vi "Blank Module Data (Constant).vi"() -> (0 "Blank Module Data":T1)   [LabVIEW 2023, in "Error Manager.lvlib" / "New Error Dialogue GUI.lvlib"]
doc: "Outputs a \"blank\" Module Data cluster. Use this to initialise the Module Data, or to reset or clear it.\n\n\"blank\" is used to mean default, empty or initial values."
uses:
  New Error Dialogue GUI.lvlib
  Module Data (cluster).ctl
  Module Data - Inputs (cluster).ctl
  Module Data - Work (cluster).ctl
  Module Data - Outputs (cluster).ctl
panel:
  # "Development\ncontrols/indicators useful for development and testing, but which are not outputs of the VI"
  # "Input\nInputs to the VI"
  # "Output\nOutputs of the VI"
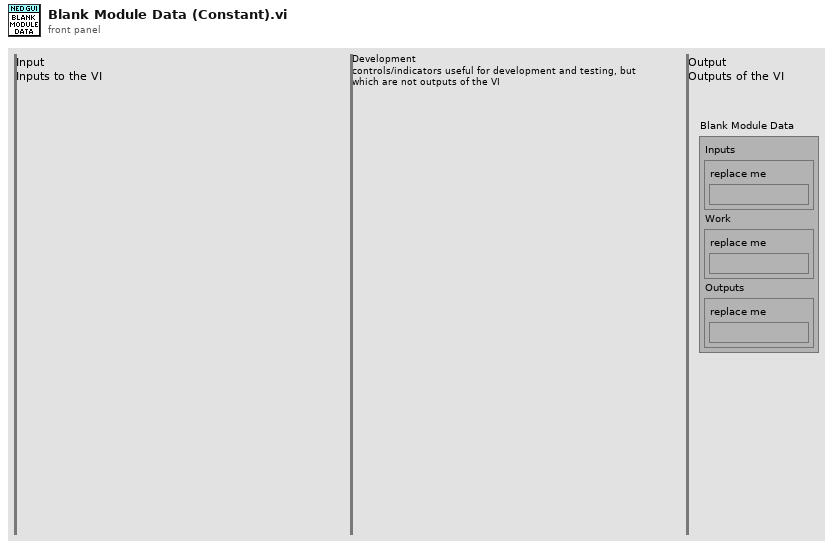
[diagram p1: front panel]
types:
  T1 = typedef "Error Manager.lvlib/New Error Dialogue GUI.lvlib/Module Data (cluster).ctl" = cluster{"Inputs":T2, "Work":T3, "Outputs":T4}
  T2 = typedef "Error Manager.lvlib/New Error Dialogue GUI.lvlib/Module Data - Inputs (cluster).ctl" = cluster{"replace me":string}
  T3 = typedef "Error Manager.lvlib/New Error Dialogue GUI.lvlib/Module Data - Work (cluster).ctl" = cluster{"replace me":string}
  T4 = typedef "Error Manager.lvlib/New Error Dialogue GUI.lvlib/Module Data - Outputs (cluster).ctl" = cluster{"replace me":string}
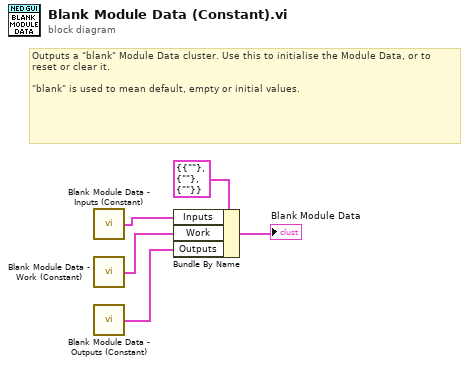
[diagram p0: block diagram]
diagram:
  # "Outputs a \"blank\" Module Data cluster. Use this to initialise the Module Data, or to reset or clear it.\n\n\"blank\" is used to mean default, empty or initial values."
  n1 = call "Blank Module Data - Inputs (Constant).vi"() -> ("Blank Module Data - Inputs"=w3:T2)
  n2 = call "Blank Module Data - Work (Constant).vi"() -> ("Blank Module Data - Work"=w2:T3)
  n3 = call "Blank Module Data - Outputs (Constant).vi"() -> ("Blank Module Data - Outputs"=w1:T4)
  n4 = Bundle By Name(cluster=T1 {"Inputs"={"replace me"=""}, "Work"={"replace me"=""}, "Outputs"={"replace me"=""}} ("Module Data"), "Inputs"=w3, "Work"=w2, "Outputs"=w1) -> (→"Blank Module Data":T1)
